vi "BangBang_AtSetpoint.vi"(11 "BANG_BANG":T1 {"Measurment" format="%13.5p"; "Setpoint" format="%13.5p"; "Tolerance" format="%13.5p"}) -> (3 "AtSetpoint":bool)   [LabVIEW 2019, in "Trajectory_Library.lvlib"]
doc: "Returns true if the error is within the tolerance of the setpoint.\n\nInput:\n - BangBang -- Data cluster\n\nOutput\n - AtSetpoint -- Returns TRUE if within error tolerance."
uses:
  Trajectory_Library.lvlib
  TypeDef/BANG_BANG.ctl
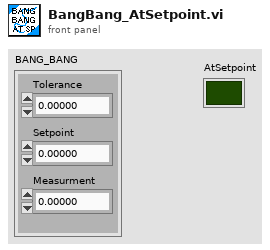
[diagram p1: front panel]
types:
  T1 = typedef "Trajectory_Library.lvlib/BANG_BANG.ctl" = cluster{"Tolerance":dbl, "Setpoint":dbl, "Measurment":dbl}
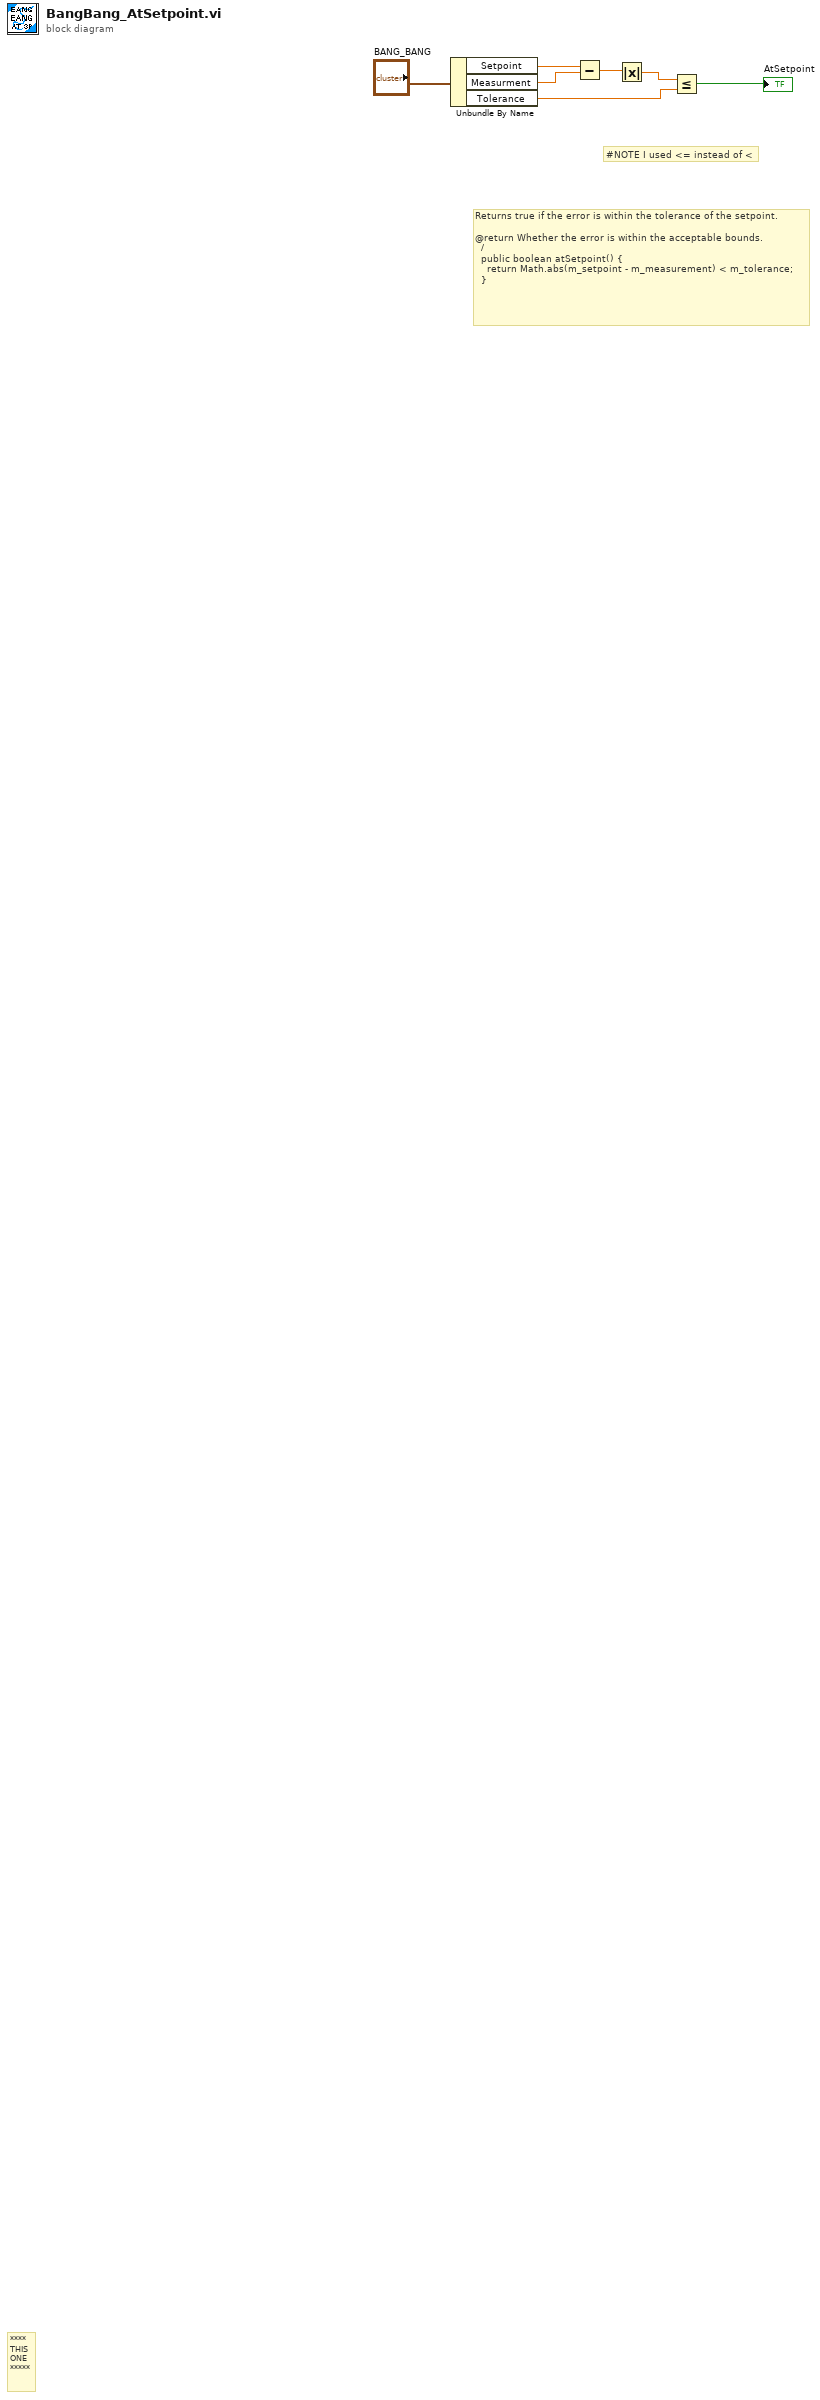
[diagram p0: block diagram]
diagram:
  # "#NOTE I used <= instead of <"
  # "Returns true if the error is within the tolerance of the setpoint.\n  \n@return Whether the error is within the acceptable bounds.\n  /\n  public boolean atSetpoint() {\n    return Math.abs(m_setpoint - m_measurement) < m_tolerance;\n  }"
  # "****\nTHIS\nONE\n*****"
  n1 = Unbundle By Name("BANG_BANG") -> ("Setpoint"=w5:dbl, "Measurment"=w4:dbl, "Tolerance"=w2:dbl)
  n2 = Subtract(x=w5, y=w4) -> (x-y=w6:dbl)
  n3 = Absolute Value(x=w6) -> (abs(x)=w3:dbl)
  n4 = Less Or Equal?(x=w3, y=w2) -> (x <= y?=→"AtSetpoint":bool)
